vi "SMS_RAMP_STATUS.vi"(0 "CRYogenic:(":errorcluster, 1 "Hulk_SMS_addr":refnum<visa-resource-name>) -> (2 "error out":errorcluster, 3 "selection":bool, 4 "read buffer":string)   [LabVIEW 2017]
uses:
  SMScontrols.ctl
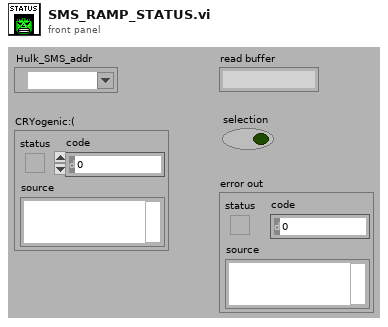
[diagram p1: front panel]
types:
  T1 = typedef "SMScontrols.ctl" = enum16{"UPDATE", "GET OUTPUT", "RAMP ZERO", "RAMP MID", "RAMP MAX", "RAMP STATUS", "PAUSE OFF", "PAUSE ON", "HEATER OFF", "HEATER ON", "TESLA OFF", "TESLA ON", "DIRECTION +", "DIRECTION -", "DIRECTION 0", "SET MID", "SET MAX", "SET RAMP", "SET LIMIT", "SET TPA", "SET HEATER"}
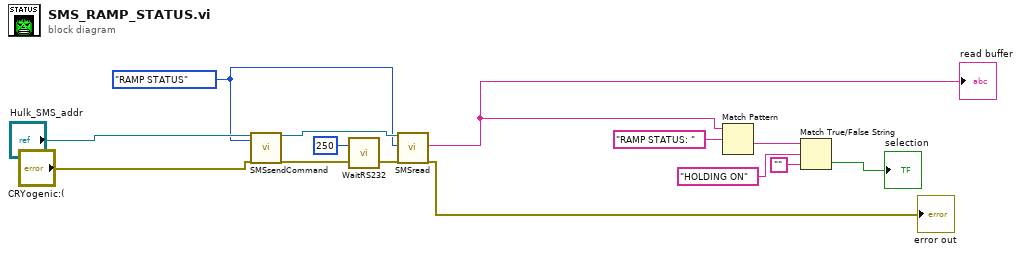
[diagram p0: block diagram]
diagram:
  w1 = SMScontrols."RAMP STATUS" ("SMS controls")
  n1 = call "SMSsendCommand.vi"("HULK SMS address in"="Hulk_SMS_addr", "SMS controls"=w1, "error in"="CRYogenic:(") -> ("HULK SMS address out"=w3:refnum<visa-resource-name>, "error out"=w5:errorcluster)  [unwired: 14 in, 1 out]
  n2 = call "WaitRS232.vi"("error in"=w5, "delay[160 ms]"=u32 250) -> ("error out"=w4:errorcluster)  [unwired: 1 in]
  n3 = call "SMSread.vi"("HULK SMS address in"=w3, "SMS controls"=w1, "error in"=w4) -> ("read buffer"=w13:string, "error out"=→"error out":errorcluster)  [unwired: 11 in, 4 out]
  "read buffer" <- w13
  n4 = Match Pattern(string=w13, regular expression="RAMP STATUS: ") -> (after substring=w11:string)  [unwired: 1 in, 3 out]
  n5 = Match True/False String(2:"", 3:"HOLDING ON" ("true string"), 4:w11) -> (0:→"selection":bool)  [unwired: 1 out]
